vi "Read Dev Average.vi"(8 "error in (no error)":errorcluster, 11 "VISA resource name":refnum<visa-resource-name>) -> (0 "error out":errorcluster, 2 "dev average":dbl, 3 "VISA resource name out":refnum<visa-resource-name>)   [LabVIEW 2025, in "Andeen-Hagerling 2700A.lvlib"]
doc: "Return the value of the deviation mode average time parameter.\n\nDeviation mode average time is minimum time interval during which\nmeasurement samples are averaged in the deviation N Data Stream \ncase or during which the occurrence of an error is watched for in the\ndeviation E Data Stream case."
uses:
  Andeen-Hagerling 2700A.lvlib
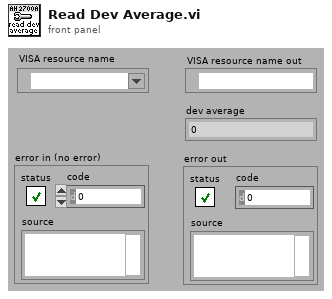
[diagram p1: front panel]
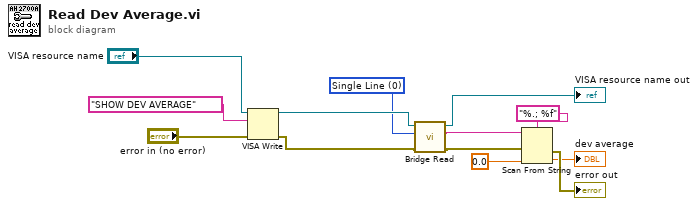
[diagram p0: block diagram]
diagram:
  w1 = u16 0 items=["Single Line", "Multi-Line"] ("Multiline")
  n1 = VISA Write(VISA resource name="VISA resource name", write buffer="SHOW DEV AVERAGE" ("command"), error in (no error)="error in (no error)") -> (VISA resource name out=w3:refnum<visa-resource-name>, error out=w2:errorcluster)  [unwired: 1 out]
  n2 = call "Bridge Read.vi"("error in (no error)"=w2, "multiline"=w1, "VISA resource name"=w3) -> ("error out"=w5:errorcluster, "read buffer"=w4:string, "VISA resource name out"=→"VISA resource name out":refnum<visa-resource-name>)  [unwired: 6 in]
  n3 = Scan From String(format string="%.; %f", input string=w4, error in=w5, default 1=0.0 ("default value 1")) -> (error out=→"error out":errorcluster, output 1=→"dev average":dbl)  [unwired: 1 in, 2 out]
